vi "Main.vi"(11 "Module Admin":refnum<class "Delacor_lib_QMH_Module Admin.lvclass">) -> ()   [LabVIEW 2020, in "Logging.lvlib"]
doc: "This template is based off of the Queued Message Handler design pattern and the Queued Message Handler project template that ships with LabVIEW.\n\nThe main difference is that the queue is private to this module and communication between modules is performed via Broadcast and Request events.\n\nRequest events are wrapped in public API methods and are handled in the Event Handling Loop (EHL) of this VI. Any module can register for Broadcast events sent by this module. The EHL generates messages based on user interface actions.\n\nThe Message Handling Loop (MHL) processes messages generated by the EHL, or by other messages. The messages are string values, so new messages can be added easily to the Message Cases case structure in the MHL. Each message cluster can also provide an optional value for Message Data, which is a variant that can be converted to whatever message-specific data is required.\n_____\nBased on Delacor QMH Project Template 6.0.0.89."
uses:
  Logging.lvlib
  <vilib>/Delacor/Delacor QMH/Libraries/Module Admin_class/Delacor_lib_QMH_Module Admin.lvclass
  Module Data--cluster.ctl
  Stop Argument--cluster.ctl
  <vilib>/Delacor/Delacor QMH/Libraries/Message Queue_class/Delacor_lib_QMH_Message Queue.lvclass/Delacor_lib_QMH_Message Queue.ctl
  <vilib>/Delacor/Delacor QMH/Libraries/Module Admin_class/Delacor_lib_QMH_Module Admin.lvclass/Delacor_lib_QMH_Module Admin.ctl
  <vilib>/Utility/miscctls.llb/LVPointTypeDef.ctl
  <vilib>/Utility/sysdir.llb/System Directory Type.ctl
  <vilib>/Delacor/Delacor QMH/Libraries/Message Queue_class/Delacor_lib_QMH_Enqueue Message (Single).vi
  <vilib>/Delacor/Delacor QMH/Libraries/Module Admin_class/Delacor_lib_QMH_Get External Launch.vi
  <vilib>/Utility/error.llb/Error Cluster From Error Code.vi
  <vilib>/ErrorRing/Error Ring.xnode
  <vilib>/Delacor/Delacor QMH/Libraries/Message Queue_class/Delacor_lib_QMH_Message Queue.lvclass
  Acquisition/Acquisition.lvlib
  Settings/Settings.lvlib
panel:
  out "TypeAcqName 2":string
  out "TypeAcqName":string
  out "error out":errorcluster
  out "Status":string
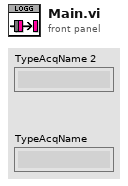
[diagram p1: front panel]
types:
  T1 = typedef "Logging.lvlib/Request Events--cluster.ctl" = cluster{"Stop Module":refnum<user-event>, "Show Panel":refnum<user-event>, "Hide Panel":refnum<user-event>, "Get Module Execution Status":refnum<user-event>, "Show Diagram":refnum<user-event>}
  T2 = typedef "Acquisition.lvlib/Broadcast Events--cluster.ctl" = cluster{"Module Did Init":refnum<user-event>, "Status Updated":refnum<user-event>, "Error Reported":refnum<user-event>, "Module Did Stop":refnum<user-event>, "Update Module Execution Status":refnum<user-event>, "AnalogDataAcquired":refnum<user-event>, "DigitalDataAcquired":refnum<user-event>, "TypeAcq":refnum<user-event>}
  T3 = typedef "Settings.lvlib/Broadcast Events--cluster.ctl" = cluster{"Module Did Init":refnum<user-event>, "Status Updated":refnum<user-event>, "Error Reported":refnum<user-event>, "Module Did Stop":refnum<user-event>, "Update Module Execution Status":refnum<user-event>, "NameTest":refnum<user-event>, "SecuenceHasBeenSent":refnum<user-event>, "TypeSignal":refnum<user-event>}
  T4 = typedef "Logging.lvlib/Module Data--cluster.ctl" = cluster{"Status":string, "TestName":string, "AnalogData":waveform(dbl)[], "TypeAcqName":string, "DigitalData":bool[]}
  T5 = enum32{"invalid lock state", "Not Locked", "Locked (No Password)", "Password-protected"}
  T6 = typedef "Logging.lvlib/Stop Argument--cluster.ctl" = cluster{"Origin":string, "Exit via Stop Module Req?":bool, "Wait for Module to stop?":bool}
  T7 = typedef "LVPointTypeDef.ctl" = cluster{"Horizontal":i16, "Vertical":i16}
  T8 = enum32{"Invalid", "Standard", "Closed", "Hidden", "Minimized", "Maximized"}
  T9 = enum16{"open", "open or create", "create or replace", "create", "open (read-only)"}
  T10 = typedef "System Directory Type.ctl" = i32
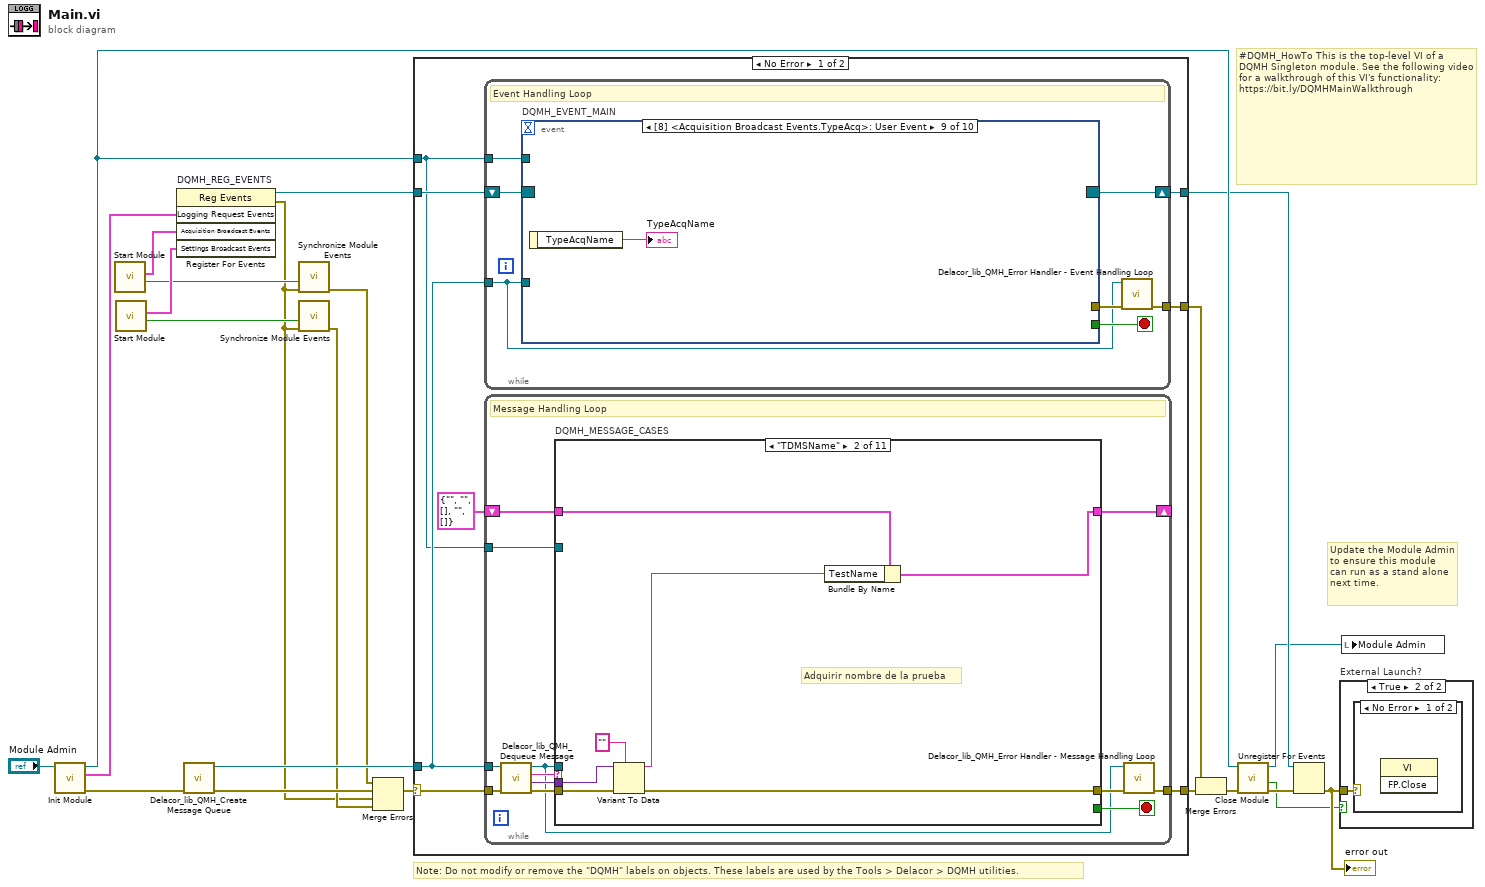
[diagram p0: block diagram]
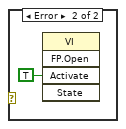
[diagram p3: hidden frame]
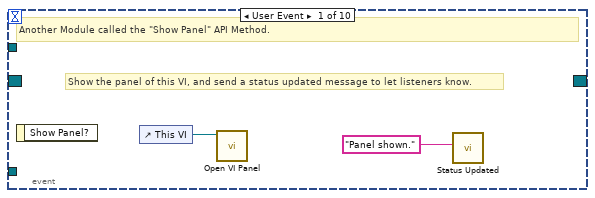
[diagram p4: hidden frame]
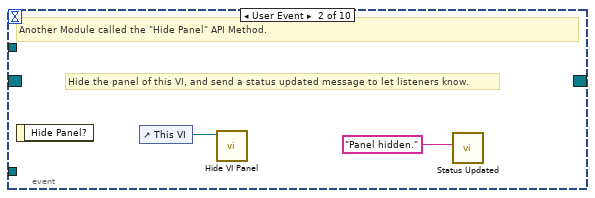
[diagram p5: hidden frame]
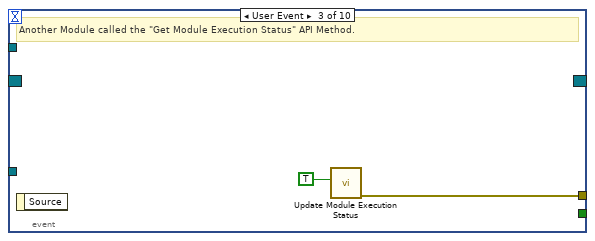
[diagram p6: hidden frame]
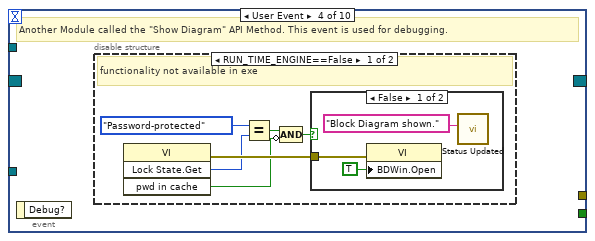
[diagram p7: hidden frame]
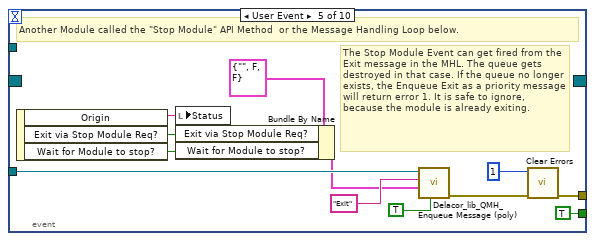
[diagram p10: hidden frame]
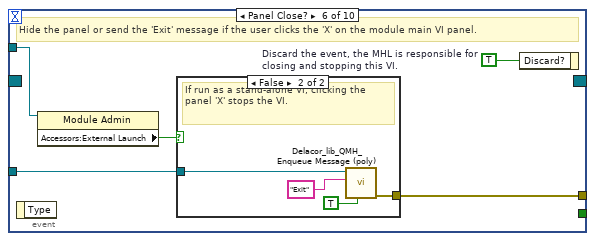
[diagram p11: hidden frame]
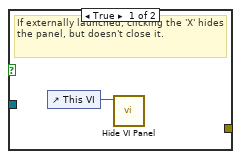
[diagram p12: hidden frame]
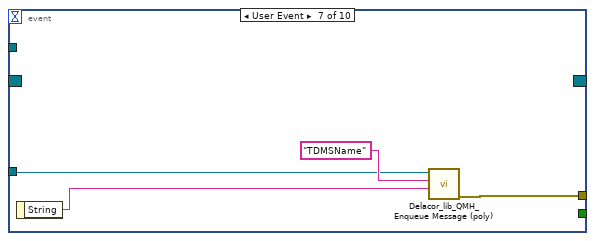
[diagram p13: hidden frame]
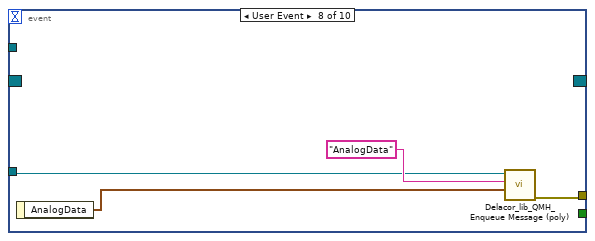
[diagram p14: hidden frame]
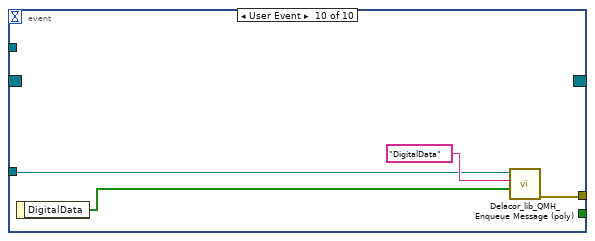
[diagram p15: hidden frame]
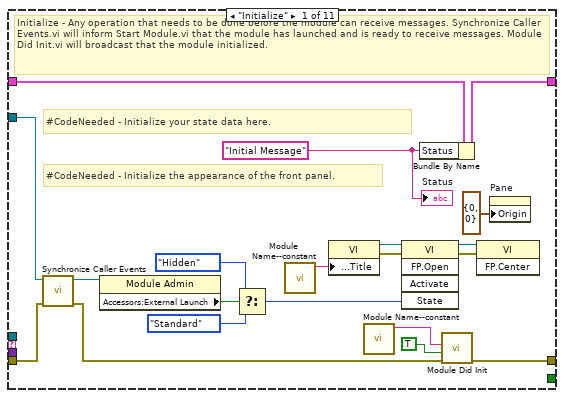
[diagram p16: hidden frame]
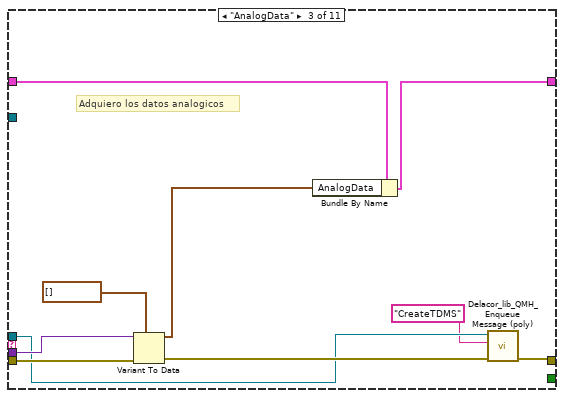
[diagram p17: hidden frame]
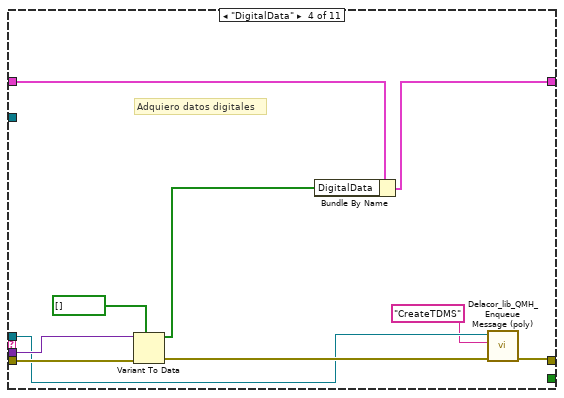
[diagram p18: hidden frame]
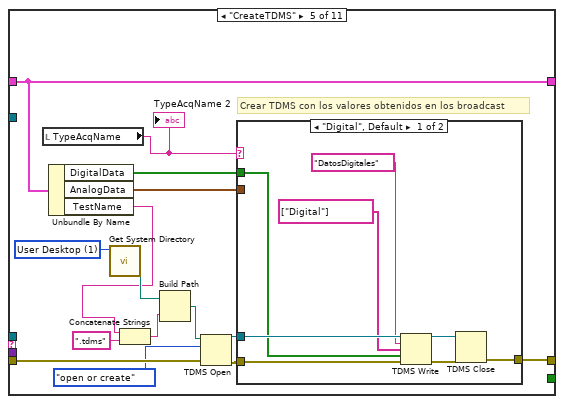
[diagram p19: hidden frame]
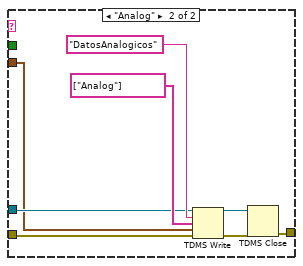
[diagram p20: hidden frame]
diagram:
  # "#DQMH_HowTo This is the top-level VI of a DQMH Singleton module. See the following video for a walkthrough of this VI's functionality: https://bit.ly/DQMHMainWalkthrough"
  # "Note: Do not modify or remove the \"DQMH\" labels on objects. These labels are used by the Tools > Delacor > DQMH utilities."
  # "Update the Module Admin to ensure this module can run as a stand alone next time."
  n1 = call "Init Module.vi"("Singleton Module Admin in"="Module Admin") -> ("error out"=w22:errorcluster, "Logging Request Events"=w12:T1, "Singleton Module Admin out"=w15:refnum<class "Delacor_lib_QMH_Module Admin.lvclass">)  [unwired: 8 in]
  n2 = call "Start Module.vi"() -> ("Wait for Event Sync?"=w3:bool, "Acquisition Broadcast Events"=w4:T2)  [unwired: 8 in, 2 out]
  n3 = call "Start Module.vi"() -> ("Wait for Event Sync?"=w6:bool, "Settings Broadcast Events"=w7:T3)  [unwired: 8 in, 2 out]
  n4 = register-events "DQMH_REG_EVENTS"(w12, w4, w7) -> (reference out=w13:refnum<event-registration>, error out=w2:errorcluster)  [unwired: 2 in]
  n5 = call <vilib>:"Delacor_lib_QMH_Create Message Queue.vi"("error in"=w22) -> ("error out"=w17:errorcluster, "Message Queue"=w11:refnum<class "Delacor_lib_QMH_Message Queue.lvclass">)  [unwired: 9 in]
  n6 = call "Synchronize Module Events.vi"("error in"=w2, "Wait for Event Sync?"=w3) -> ("error out"=w1:errorcluster)  [unwired: 9 in]
  n7 = call "Synchronize Module Events.vi"("error in"=w2, "Wait for Event Sync?"=w6) -> ("error out"=w5:errorcluster)  [unwired: 9 in]
  n8 = Merge Errors(w1, w17, w2, w5) -> (w16:errorcluster)
  n9 = case shown="No Error" w16 {
    selector: w16 -> [w29 w233]
    tunnel: [w31 w232] -> w23
    tunnel: [w28 w238] -> w14
    tunnel: w13 -> [w26 w238]
    tunnel: w11 -> [w25 w231]
    tunnel: [w30 _] -> w20
    tunnel: w15 -> [w24 w234]
    frame No Error {
      n10 = while {
        tunnel: w25 -> [w32]
        shift-right: [w35] -> w28
        shift-left: w26 -> [w36]
        tunnel: [w37] -> w30
        tunnel: w24 -> [w33]
        stop <- w34 stop-if-true
        # "Event Handling Loop"
        n11 = event "DQMH_EVENT_MAIN" shown="[8] <Acquisition Broadcast Events.TypeAcq>: User Event" {
          selector: w36 -> [_ _ _ _ _ _ _ _ _ _]
          dyn-events: [_ _ _ _ _ _ _ _ _ _] -> w35
          timeout: _ -> [_ _ _ _ _ _ _ _ _ _]
          tunnel: [_ _ _ _ TRUE ("Discard?") _ _ _ _ _] -> w34
          tunnel: w32 -> [_ _ _ _ w61 w68 w77 w81 _ w86]
          tunnel: [_ _ w44 _ w64 w70 w78 w82 _ w87] -> w38
          tunnel: w33 -> [_ _ _ _ _ w67 _ _ _ _]
          event User Event {
            # "Show the panel of this VI, and send a status updated message to let listeners know."
            # "Another Module called the \"Show Panel\" API Method."
            n12 = event-data() -> ()  [unwired: 1 in, 1 out]
            n13 = control-ref of="This VI"() -> (w40:refnum<vi>)
            n14 = call "Open VI Panel.vi"("VI"=w40) -> ()  [unwired: 10 in, 1 out]
            n15 = call "Status Updated.vi"("Status"="Panel shown." ("format string")) -> ()  [unwired: 10 in, 1 out]
          }
          event User Event {
            # "Hide the panel of this VI, and send a status updated message to let listeners know."
            # "Another Module called the \"Hide Panel\" API Method."
            n16 = event-data() -> ()  [unwired: 1 in, 1 out]
            n17 = control-ref of="This VI"() -> (w42:refnum<vi>)
            n18 = call "Hide VI Panel.vi"("VI"=w42) -> ()  [unwired: 10 in, 1 out]
            n19 = call "Status Updated.vi"("Status"="Panel hidden." ("format string")) -> ()  [unwired: 10 in, 1 out]
          }
          event User Event {
            # "Another Module called the \"Get Module Execution Status\" API Method."
            n20 = event-data() -> ()  [unwired: 1 in, 1 out]
            n21 = call "Update Module Execution Status.vi"("Running?"=TRUE) -> ("error out"=w44:errorcluster)  [unwired: 10 in]
          }
          event User Event {
            # "Another Module called the \"Show Diagram\" API Method. This event is used for debugging."
            n22 = event-data() -> ()  [unwired: 1 in, 1 out]
            n23 = disable-structure shown="RUN_TIME_ENGINE==False" {
              frame condition #0 (active) {
                # "functionality not available in exe"
                n24 = invoke class="VI" method="Lock State.Get"() -> (error out=w50:errorcluster, "Get Lock State"=w49:T5, "pwd in cache"=w46:bool)  [unwired: 4 in, 1 out]
                n25 = Equal?(x=T5."Password-protected", y=w49) -> (x = y?=w47:bool)
                n26 = Compound Arithmetic op=AND(w47, invert w46) -> (w45:bool)
                n27 = case shown="False" w45 {
                  tunnel: w50 -> [w53 _]
                  frame False {
                    n28 = property class="VI"(error in=w53, "BDWin.Open"=TRUE ("Block Diagram Window:Open")) -> ()  [unwired: 1 in, 2 out]
                    n29 = call "Status Updated.vi"("Status"="Block Diagram shown." ("format string")) -> ()  [unwired: 10 in, 1 out]
                  }
                  frame True {
                    # "Password-protected VI, and the password is not in the cache. Do not show the diagram."
                  }
                }
              }
              frame condition #1 {
              }
            }
          }
          event User Event {
            # "The Stop Module Event can get fired from the Exit message in the MHL. The queue gets destroyed in that case. If the queue no longer exists, the Enqueue Exit as a priority message will return error 1. It is safe to ignore, because the module is already exiting."
            # "Another Module called the \"Stop Module\" API Method  or the Message Handling Loop below."
            n30 = event-data() -> ("Origin"=w60:string, "Exit via Stop Module Req?"=w56:bool, "Wait for Module to stop?"=w55:bool)  [unwired: 1 in]
            n31 = local write "Status"(w60) -> ()
            n32 = Bundle By Name(cluster=T6 {"Origin"="", "Exit via Stop Module Req?"=FALSE, "Wait for Module to stop?"=FALSE} ("Stop Argument"), "Exit via Stop Module Req?"=w56, "Wait for Module to stop?"=w55) -> (w54:T6)
            n33 = call-poly <vilib>:"Delacor_lib_QMH_Enqueue Message (poly).vi"("Priority Message? (F)"=TRUE, "Message Data"=w54, "Message"="Exit", "Message Queue in"=w61) -> ("error out"=w65:errorcluster)  [unwired: 6 in, 1 out]
            n34 = call <vilib>:"Clear Errors.vi"("error in (no error)"=w65, "specific error code to clear (0: all)"=1) -> ("error out"=w64:errorcluster)  [unwired: 4 in, 1 out]
          }
          event Panel Close? {
            w69 = TRUE  # Discard the event, the MHL is responsible for closing and stopping this VI.
            # "Hide the panel or send the 'Exit' message if the user clicks the 'X' on the module main VI panel."
            n35 = event-data() -> ()  [unwired: 1 in, 1 out]
            n36 = property class="Module Admin"(reference=w67) -> ("Accessors:External Launch"=w66:bool)  [unwired: 1 in, 2 out]
            n37 = case shown="False" w66 {
              tunnel: w68 -> [_ w74]
              tunnel: [_ w75] -> w70
              frame True {
                # "If externally launched, clicking the 'X' hides the panel, but doesn't close it."
                n38 = control-ref of="This VI"() -> (w71:refnum<vi>)
                n39 = call "Hide VI Panel.vi"("VI"=w71) -> ()  [unwired: 10 in, 1 out]
              }
              frame False {
                # "If run as a stand-alone VI, clicking the panel 'X' stops the VI."
                n40 = call-poly <vilib>:"Delacor_lib_QMH_Enqueue Message (poly).vi"("Priority Message? (F)"=TRUE, "Message"="Exit", "Message Queue in"=w74) -> ("error out"=w75:errorcluster)  [unwired: 7 in, 1 out]
              }
            }
            n41 = event-data("Discard?"=w69) -> ()  [unwired: 1 in, 1 out]
          }
          event User Event {
            n42 = event-data() -> ("String"=w76:string)  [unwired: 1 in]
            n43 = call-poly <vilib>:"Delacor_lib_QMH_Enqueue Message (poly).vi"("Message Data"=w76, "Message"="TDMSName", "Message Queue in"=w77) -> ("error out"=w78:errorcluster)  [unwired: 7 in, 1 out]
          }
          event User Event {
            n44 = event-data() -> ("AnalogData"=w80:waveform(dbl)[])  [unwired: 1 in]
            n45 = call-poly <vilib>:"Delacor_lib_QMH_Enqueue Message (poly).vi"("Message Data"=w80, "Message"="AnalogData", "Message Queue in"=w81) -> ("error out"=w82:errorcluster)  [unwired: 7 in, 1 out]
          }
          event User Event {
            n46 = event-data() -> ("TypeAcqName"=→"TypeAcqName":string)  [unwired: 1 in]
          }
          event User Event {
            n47 = event-data() -> ("DigitalData"=w85:bool[])  [unwired: 1 in]
            n48 = call-poly <vilib>:"Delacor_lib_QMH_Enqueue Message (poly).vi"("Message Data"=w85, "Message"="DigitalData", "Message Queue in"=w86) -> ("error out"=w87:errorcluster)  [unwired: 7 in, 1 out]
          }
        }
        n49 = call-dynamic "Delacor_lib_QMH_Error Handler - Event Handling Loop.vi"("error in"=w38, "Message Queue in"=w32) -> ("dup error in"=w37:errorcluster)  [unwired: 8 in, 1 out]
      }
      n50 = while {
        tunnel: w25 -> [w91]
        shift-right: [w95] -> _
        shift-left: T4 {"Status"="", "TestName"="", "AnalogData"=[], "TypeAcqName"="", "DigitalData"=[]} ("Data Cluster") -> [w96]
        tunnel: w29 -> [w99]
        tunnel: [w97] -> w31
        tunnel: w24 -> [w89]
        stop <- w94 stop-if-true
        # "Message Handling Loop"
        n51 = call-dynamic "Delacor_lib_QMH_Dequeue Message.vi"("error in"=w99, "Message Queue in"=w91) -> ("error out"=w98:errorcluster, "Message Data"=w92:variant, "Message"=w93:string, "Message Queue out"=w90:refnum<class "Delacor_lib_QMH_Message Queue.lvclass">)  [unwired: 6 in]
        n52 = case "DQMH_MESSAGE_CASES" shown="\"TDMSName\"" w93 {
          selector: w93 -> [_ _ _ _ _ _ _ _ _ _ w218]
          tunnel: w90 -> [_ _ w133 w143 _ _ _ _ w188 w210 _]
          tunnel: w98 -> [w118 w127 w137 w147 w160 w180 w183 w185 w195 w216 w220]
          tunnel: [w116 w121 w136 w146 w158 w180 w182 w185 w191 w213 w221] -> w100
          tunnel: w96 -> [w107 w124 w131 w141 w162 w179 w181 w184 w190 w209 w219]
          tunnel: [w106 w123 w130 w140 w162 w179 w181 w184 w190 w209 w219] -> w95
          tunnel: [_ _ _ _ _ _ _ _ _ w208 _] -> w94
          tunnel: w92 -> [_ w126 w134 w144 _ _ _ _ w189 w207 _]
          tunnel: w89 -> [w108 _ _ _ _ _ _ _ w187 w202 _]
          frame "Initialize" {
            w102 = "Initial Message" ("Initial Message")
            # "#CodeNeeded - Initialize the appearance of the front panel."
            # "#CodeNeeded - Initialize your state data here."
            # "Initialize - Any operation that needs to be done before the module can receive messages. Synchronize Caller Events.vi will inform Start Module.vi that the module has launched and is ready to receive messages. Module Did Init.vi will broadcast that the module initialized."
            n53 = call "Synchronize Caller Events.vi"("error in (no error)"=w118, "Singleton Module Admin in"=w108) -> ("error out"=w117:errorcluster, "Singleton Module Admin out"=w103:refnum<class "Delacor_lib_QMH_Module Admin.lvclass">)  [unwired: 8 in]
            n54 = property class="Module Admin"(reference=w103) -> ("Accessors:External Launch"=w112:bool)  [unwired: 1 in, 2 out]
            n55 = Select(t=T8."Hidden" ("State"), s=w112, f=T8."Standard" ("State")) -> (s? t:f=w109:T8)
            n56 = call "Module Name--constant.vi"() -> ("Module Name"=w115:string)  [unwired: 11 in]
            n57 = property class="VI"("Front Panel.Title"=w115) -> (reference out=w114:refnum<vi>, error out=w120:errorcluster)  [unwired: 2 in]
            n58 = call "Module Name--constant.vi"() -> ("Module Name"=w104:string)  [unwired: 11 in]
            n59 = invoke class="VI" method="FP.Open"(reference=w114, error in=w120, "State"=w109) -> (reference out=w113:refnum<vi>, error out=w119:errorcluster)  [unwired: 2 in, 3 out]
            n60 = Bundle By Name(cluster=w107, "Status"=w102) -> (w106:T4)
            n61 = call "Module Did Init.vi"("error in (no error)"=w117, "Initialized?"=TRUE, "Origin"=w104) -> ("error out"=w116:errorcluster)  [unwired: 8 in]
            n62 = invoke class="VI" method="FP.Center"(reference=w113, error in=w119) -> ()  [unwired: 1 in, 3 out]
            n63 = property on="Pane" class="Pane"("Origin"=T7 {"Horizontal"=0, "Vertical"=0}) -> ()  [unwired: 2 in, 2 out]
            "Status" <- w102
          }
          frame "TDMSName" {
            # "Adquirir nombre de la prueba"
            n64 = Variant To Data(error in=w127, type="", Variant=w126) -> (data=w122:string, error out=w121:errorcluster)
            n65 = Bundle By Name(cluster=w124, "TestName"=w122) -> (w123:T4)
          }
          frame "AnalogData" {
            # "Adquiero los datos analogicos"
            n66 = Variant To Data(error in=w137, type=waveform(dbl)[] [] ("AnalogData"), Variant=w134) -> (data=w128:waveform(dbl)[], error out=w135:errorcluster)
            n67 = Bundle By Name(cluster=w131, "AnalogData"=w128) -> (w130:T4)
            n68 = call-poly <vilib>:"Delacor_lib_QMH_Enqueue Message (poly).vi"("error in"=w135, "Message"="CreateTDMS", "Message Queue in"=w133) -> ("error out"=w136:errorcluster)  [unwired: 7 in, 1 out]
          }
          frame "DigitalData" {
            # "Adquiero datos digitales"
            n69 = Variant To Data(error in=w147, type=bool[] [] ("DigitalData"), Variant=w144) -> (data=w139:bool[], error out=w145:errorcluster)
            n70 = Bundle By Name(cluster=w141, "DigitalData"=w139) -> (w140:T4)
            n71 = call-poly <vilib>:"Delacor_lib_QMH_Enqueue Message (poly).vi"("error in"=w145, "Message"="CreateTDMS", "Message Queue in"=w143) -> ("error out"=w146:errorcluster)  [unwired: 7 in, 1 out]
          }
          frame "CreateTDMS" {
            w155 = T10 1 items=["User Home"=0, "User Desktop"=1, "User Documents"=2, "User Application Data"=3, "User Preferences"=4, "User Temporary"=5, "Public Documents"=6, "Public Application Data"=7, "Public Preferences"=8, "Public Cache"=13, "System Core Libraries"=9, "System Installed Libraries"=10, "Application Files"=11, "Boot Volume Root"=12] ("system directory type")
            # "Crear TDMS con los valores obtenidos en los broadcast"
            n72 = local read "TypeAcqName"() -> (w148:string)
            "TypeAcqName 2" <- w148
            n73 = Unbundle By Name(w162) -> ("DigitalData"=w151:bool[], "AnalogData"=w150:waveform(dbl)[], "TestName"=w152:string)
            n74 = call <vilib>:"Get System Directory.vi"("system directory type"=w155) -> ("system directory"=w157:path)  [unwired: 10 in]
            n75 = Concatenate Strings(w152, ".tdms" ("string")) -> (w154:string)
            n76 = Build Path(base path=w157, name or relative path=w154) -> (appended path=w161:path)
            n77 = TDMS Open(8:w160, 10:T9."open or create" ("operation (0:open)"), 11:w161) -> (0:w159:errorcluster, 3:w149:refnum<k34>)  [unwired: 4 in]
            n78 = case shown="\"Digital\", Default" w148 {
              tunnel: w159 -> [w170 w174]
              tunnel: [w169 w175] -> w158
              tunnel: w151 -> [w164 _]
              tunnel: w150 -> [_ w172]
              tunnel: w149 -> [w167 w173]
              frame "Digital", Default {
                n79 = TDMS Write(0:w167, 5:"DatosDigitales" ("group name in (Untitled)"), 7:string[] ["Digital"] ("channel name(s) in (Untitled)"), 9:w164, 11:w170) -> (4:w163:refnum<k34>, 15:w168:errorcluster)  [unwired: 1 in, 2 out]
                n80 = TDMS Close(8:w168, 11:w163) -> (0:w169:errorcluster)  [unwired: 1 out]
              }
              frame "Analog" {
                n81 = TDMS Write(0:w173, 5:"DatosAnalogicos" ("group name in (Untitled)"), 7:string[] ["Analog"] ("channel name(s) in (Untitled)"), 9:w172, 11:w174) -> (4:w171:refnum<k34>, 15:w178:errorcluster)  [unwired: 1 in, 2 out]
                n82 = TDMS Close(8:w178, 11:w171) -> (0:w175:errorcluster)  [unwired: 1 out]
              }
            }
          }
          frame "---Module Specific---" {
            # "Separator -- The following cases handle messages specific to this Module."
          }
          frame "---Copy This Frame---" {
            # "Duplicate this frame when creating new messages.  Change this comment in the duplicated frame to describe this message."
            n83 = Merge Errors(w183) -> (w182:errorcluster)
          }
          frame "---Exit and Error Handling---" {
            # "Separator - The following cases handle errors and exit messages."
          }
          frame "Error" {
            # "#CodeRecommended - If you ever change the name of this \"Error\" message, you'll need to update the name in the Check Loop Error.vi as well."
            # "#CodeRecommended - If the module is running in standalone mode (External Launch = FALSE), this code will pop up an error dialog and call the 'Exit' message if an error occurs. Add more fine-grained error handling here."
            # "Error - Check the error message data and respond accordingly. This message is sent by the \"Error Handler\" VIs at the end of each loop in this application."
            n84 = property class="Module Admin"(reference=w187) -> ("Accessors:External Launch"=w186:bool)  [unwired: 1 in, 2 out]
            n85 = Variant To Data(error in=w195, type=errorcluster {"status"=FALSE, "code"=0, "source"=""} ("error constant"), Variant=w189) -> (data=w196:errorcluster, error out=w193:errorcluster)
            n86 = call "Error Reported.vi"("Error"=w196) -> ()  [unwired: 10 in, 1 out]
            n87 = case shown="False" w186 {
              tunnel: [w201 _] -> w192
              tunnel: w188 -> [w199 _]
              tunnel: w196 -> [w200 _]
              frame False {
                # "If the module is running standalone, then pop up an error dialog and call the \"Exit\" message."
                n88 = call <vilib>:"Simple Error Handler.vi"("error in (no error)"=w200) -> ()  [unwired: 4 in, 5 out]
                n89 = call-poly <vilib>:"Delacor_lib_QMH_Enqueue Message (poly).vi"("Priority Message? (F)"=TRUE, "Message"="Exit", "Message Queue in"=w199) -> ("error out"=w201:errorcluster)  [unwired: 7 in, 1 out]
              }
              frame True {
                # "If the module was launched externally, calling the Error Reported broadcast VI is the only action performed by the \"Error\" message. The module's caller can then process the error appropriately."
              }
            }
            n90 = Merge Errors(w193, w192) -> (w191:errorcluster)
            n91 = local write "error out"(w191) -> ()
          }
          frame "Exit" {
            w206 = 91  # 91: not all Exit messages will have an argument
            w208 = TRUE  # Stop the VI
            # "Release the message queue reference"
            # "#CodeNeeded - Add any required cleanup code here"
            # "Exit - Exit the application."
            n92 = Variant To Data(error in=w216, type=T6 {"Origin"="", "Exit via Stop Module Req?"=FALSE, "Wait for Module to stop?"=FALSE} ("Stop Argument"), Variant=w207) -> (data=w204:T6, error out=w212:errorcluster)
            n93 = call <vilib>:"Clear Errors.vi"("error in (no error)"=w212, "specific error code to clear (0: all)"=w206) -> ("error out"=w215:errorcluster)  [unwired: 4 in, 1 out]
            n94 = control-ref of="This VI"() -> (w203:refnum<vi>)
            n95 = call-dynamic "Delacor_lib_QMH_Release Message Queue.vi"("error in"=w215, "Message Queue"=w210) -> ("error out"=w214:errorcluster)  [unwired: 9 in]
            n96 = call "Handle Exit.vi"("Stop Argument"=w204, "Admin in"=w202, "VI reference"=w203) -> ("error out"=w211:errorcluster)  [unwired: 7 in, 1 out]
            n97 = Merge Errors(w214, w211) -> (w213:errorcluster)
            n98 = call "Stop Module.vi"() -> ()  [unwired: 11 in, 1 out]
            n99 = call "Stop Module.vi"() -> ()  [unwired: 11 in, 1 out]
          }
          frame Default {
            # "'Default' case only runs if there is a message that isn't defined in any of the other cases.  Output a programming error."
            n100 = call "Module Name--constant.vi"() -> ("Module Name"=w217:string)  [unwired: 11 in]
            n101 = xnode "Error Ring"("parameter 0"=w218, "parameter 1"=w217) -> ("error out"=w222:errorcluster)
            n102 = Merge Errors(w220, w222) -> (w221:errorcluster)
          }
        }
        n103 = call-dynamic "Delacor_lib_QMH_Error Handler - Message Handling Loop.vi"("error in"=w100, "Message Queue in"=w90) -> ("dup error in"=w97:errorcluster)  [unwired: 8 in, 1 out]
      }
    }
    frame Error {
      # "Synchronize Caller Events.vi will inform Start Module.vi that the module has launched and will let the code calling Start Module.vi register for broadcasts and would permit the caller receive the broadcast that an error occurred at launch time."
      n104 = call-dynamic "Delacor_lib_QMH_Release Message Queue.vi"("error in"=w233, "Message Queue"=w231) -> ("error out"=w232:errorcluster)  [unwired: 9 in]
      n105 = call "Synchronize Caller Events.vi"("Singleton Module Admin in"=w234) -> ("error out"=w239:errorcluster)  [unwired: 9 in, 1 out]
      n106 = call "Module Name--constant.vi"() -> ("Module Name"=w237:string)  [unwired: 11 in]
      n107 = Format Into String(format string="An error occurred during initialization. %s is no longer running.", w237) -> (resulting string=w235:string)  [unwired: 2 in, 1 out]
      n108 = Merge Errors(w232, w239) -> (w240:errorcluster)
      n109 = call "Stop Module.vi"() -> ()  [unwired: 11 in, 1 out]
      n110 = call "Stop Module.vi"() -> ()  [unwired: 11 in, 1 out]
      n111 = call "Error Reported.vi"("Additional Information"=w235, "Error"=w240) -> ()  [unwired: 9 in, 1 out]
    }
  }
  n112 = Merge Errors(w20, w23) -> (w19:errorcluster)
  n113 = call "Close Module.vi"("error in (no error)"=w19, "Module Admin in"=w15) -> ("error out"=w21:errorcluster, "External Launch"=w8:bool, "Module Admin out"=w9:refnum<class "Delacor_lib_QMH_Module Admin.lvclass">)  [unwired: 7 in]
  n114 = Unregister For Events(event registration refnum=w14, error in=w21) -> (error out=w18:errorcluster)
  "error out" <- w18
  n115 = case "External Launch?" shown="True" w8 {
    tunnel: w18 -> [_ w241]
    frame False {
    }
    frame True {
      n116 = case shown="No Error" w241 {
        frame No Error {
          n117 = invoke class="VI" method="FP.Close"() -> ()  [unwired: 3 in, 3 out]
        }
        frame Error {
          n118 = invoke class="VI" method="FP.Open"("Activate"=TRUE ("Activate?")) -> ()  [unwired: 4 in, 5 out]
        }
      }
    }
  }
  n119 = local write "Module Admin"(w9) -> ()
